vi "ArduinoOpen.vi"(2 "error in (no error)":errorcluster, 3 "VISA resource name in":refnum<visa-resource-name>="COM24") -> (0 "error out":errorcluster, 1 "VISA resource name out":refnum<visa-resource-name>)   [LabVIEW 2013, in "ArduinoControl.lvclass"]
uses:
  ArduinoControl.lvclass
  <vilib>/Instr/_visa.llb/VISA Configure Serial Port (Instr).vi
panel:
  out "Moin, moin!":string
  # "Arduino Uno Edgesense"
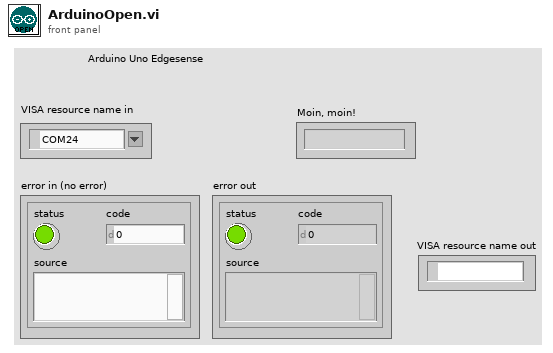
[diagram p1: front panel]
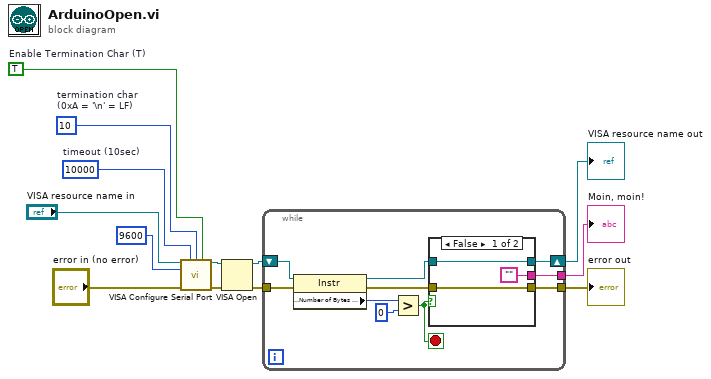
[diagram p0: block diagram]
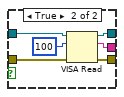
[diagram p2: hidden frame]
diagram:
  w10 = u8 10  # termination char (0xA = '\n' = LF)
  w11 = TRUE  # Enable Termination Char (T)
  w12 = u32 10000  # timeout (10sec)
  n1 = call-poly "VISA Configure Serial Port"("VISA resource name"="VISA resource name in", "timeout (10sec)"=w12, "termination char\n(0xA = '\\n' = LF)"=w10, "Enable Termination\nChar (T)"=w11, "baud rate (9600)"=9600, "error in (no error)"="error in (no error)") -> ("VISA resource name out"=w8:refnum<visa-resource-name>, "error out"=w2:errorcluster)  [unwired: 8 in]
  n2 = VISA Open(error in (no error)=w2, VISA resource name=w8) -> (VISA resource name=w6:refnum<visa-resource-name>, error out=w1:errorcluster)  [unwired: 3 in]
  n3 = while {
    shift-right: [w18] -> w5
    shift-left: w6 -> [w21]
    tunnel: [w17] -> w4
    tunnel: [w16] -> w3
    tunnel: w1 -> [w15]
    stop <- w19 stop-if-true
    n4 = property class="Instr"(reference=w21, error in=w15) -> (reference out=w20:refnum<visa-resource-name>, error out=w14:errorcluster, "Serial Settings:Number of Bytes at Serial Port"=w23:u32)
    n5 = Greater?(x=w23, y=0) -> (0:w19:bool)
    n6 = case shown="False" w19 {
      tunnel: w20 -> [w26 w32]
      tunnel: [w26 w31] -> w18
      tunnel: [w24 w30] -> w17
      tunnel: ["" w29] -> w16
      tunnel: w14 -> [w24 w28]
      frame False {
      }
      frame True {
        n7 = VISA Read(VISA resource name=w32, byte count=100, error in (no error)=w28) -> (VISA resource name out=w31:refnum<visa-resource-name>, read buffer=w29:string, error out=w30:errorcluster)  [unwired: 1 out]
      }
    }
  }
  "error out" <- w4
  "VISA resource name out" <- w5
  "Moin, moin!" <- w3
